vi "IDEX FGV.vi"(7 "Function":T2(ring), 8 "error in":errorcluster, 9 "Command":string, 10 "Position":T1(ring), 11 "VISA resource name":refnum<visa-resource-name>) -> (0 "error out":errorcluster, 3 "Read String":string)   [LabVIEW 2019, in "IDEX.lvlib"]
uses:
  IDEX.lvlib
  <vilib>/Instr/_visa.llb/VISA Configure Serial Port (Instr).vi
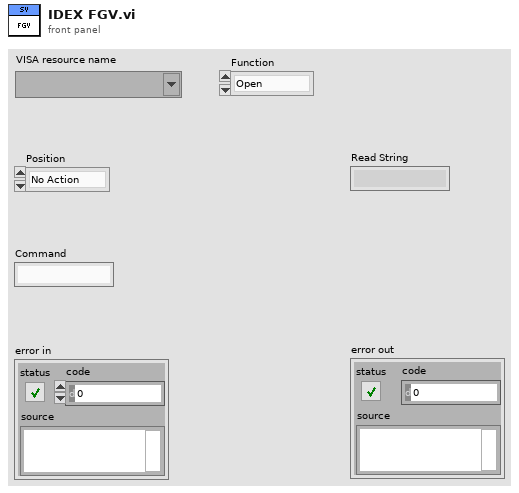
[diagram p1: front panel]
types:
  T1 = enum16{"No Action", "Position 1", "Position 2", "Position 3", "Position 4", "Position 5", "Position 6"}
  T2 = enum16{"Open", "Read", "Move", "Home", "Command", "Close"}
  T3 = cluster{"VISA resource":refnum<visa-resource-name>, "Read String":string}
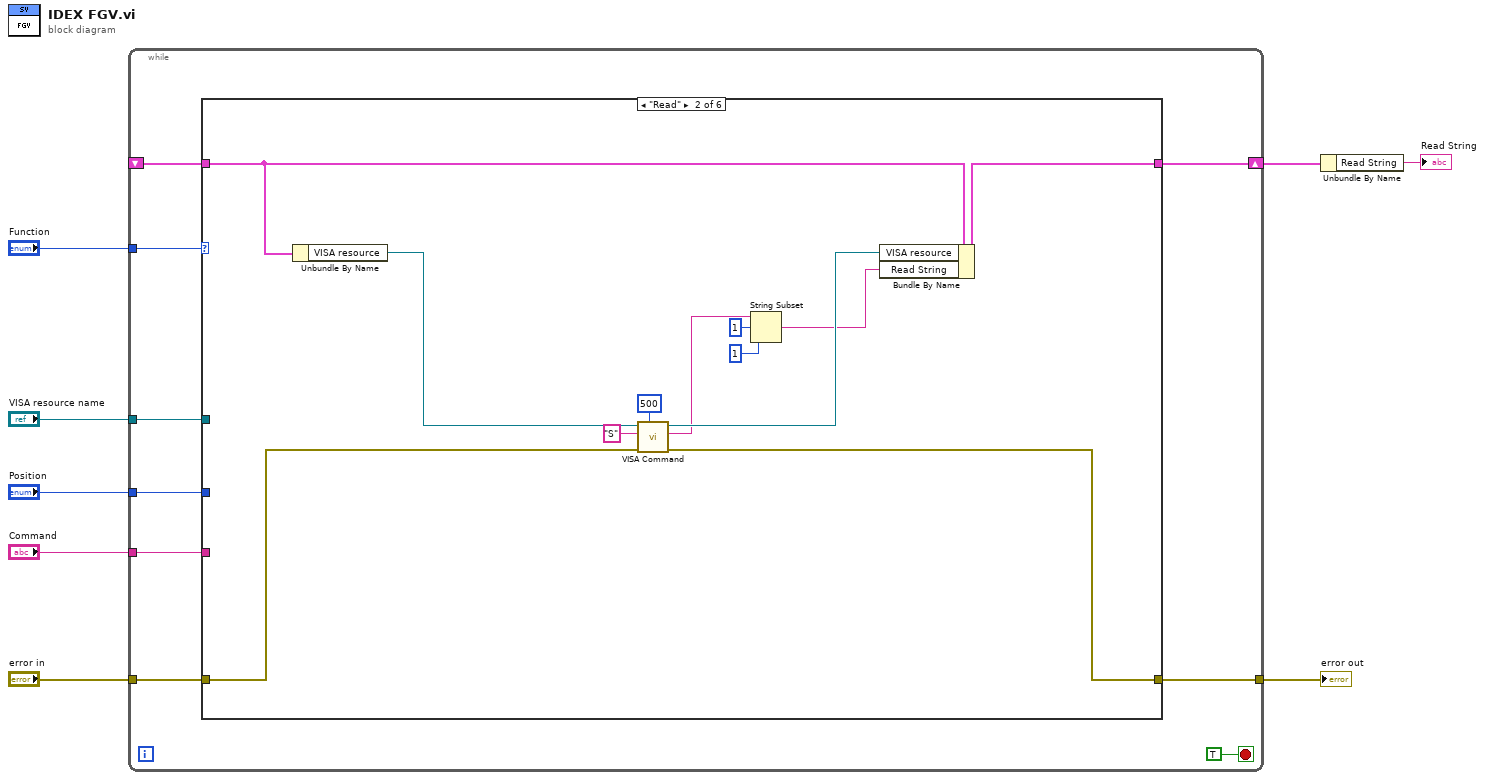
[diagram p0: block diagram]
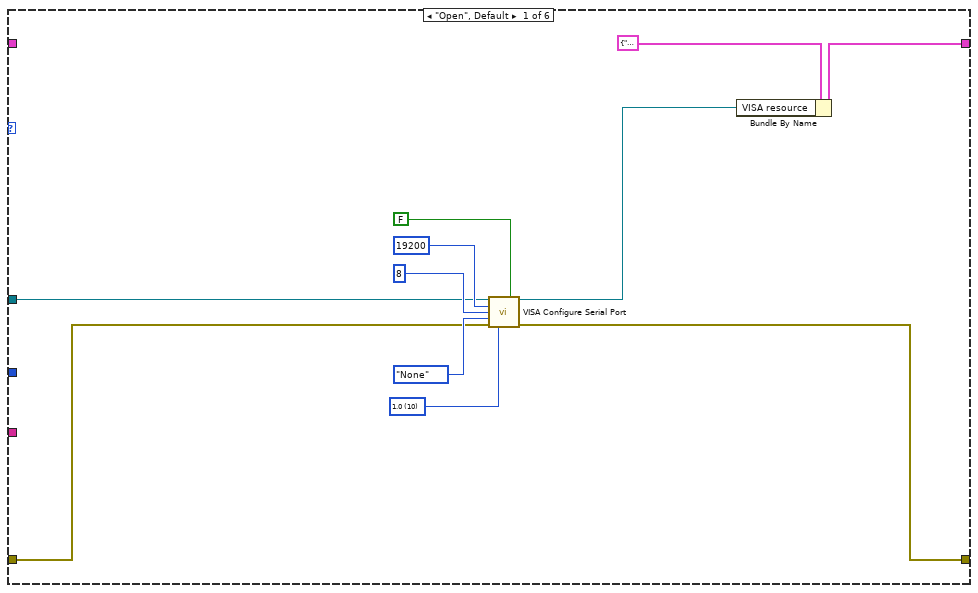
[diagram p2: hidden frame]
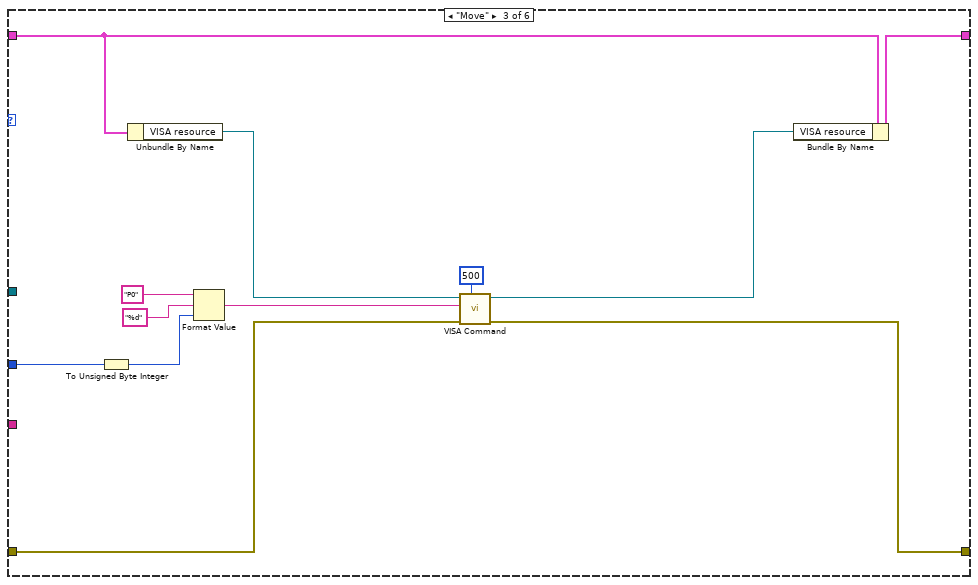
[diagram p3: hidden frame]
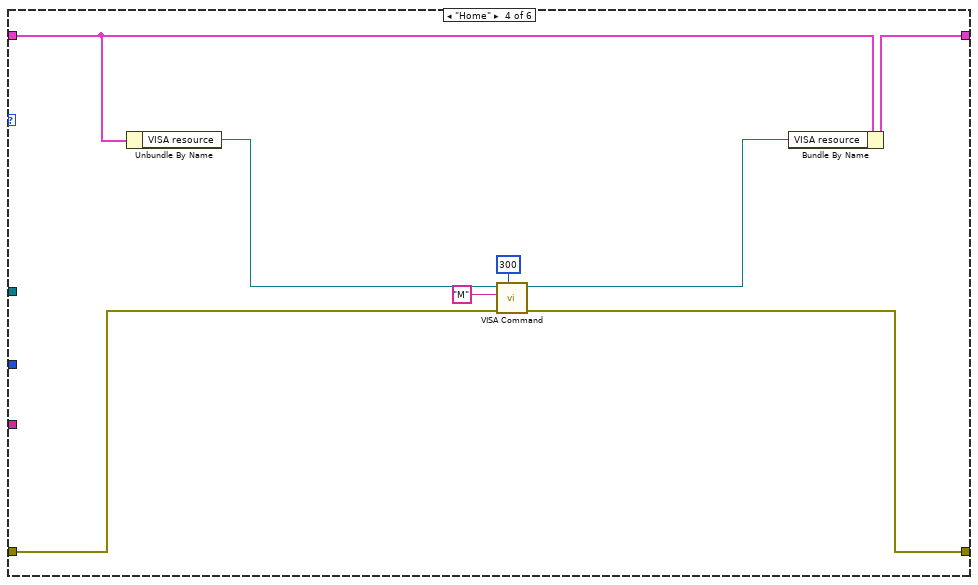
[diagram p4: hidden frame]
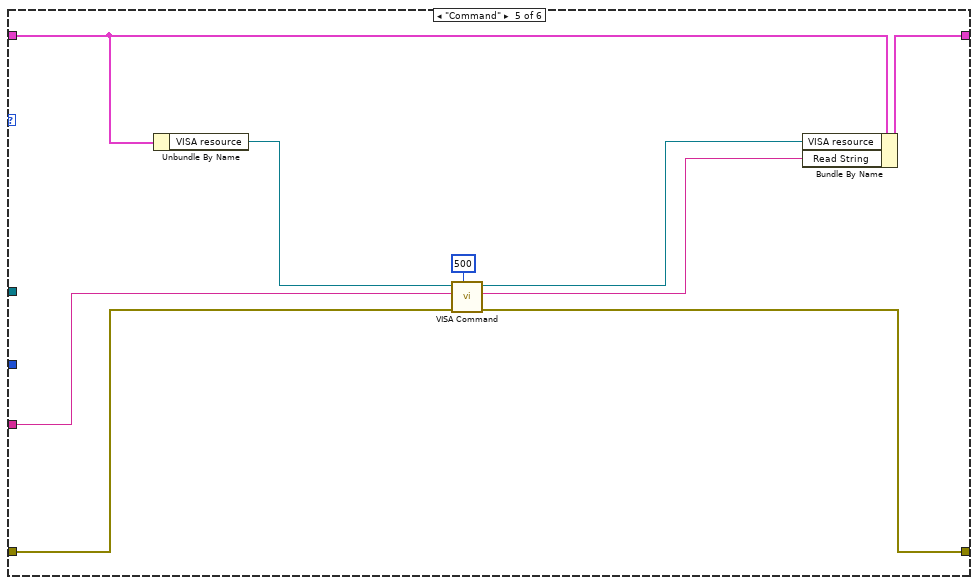
[diagram p5: hidden frame]
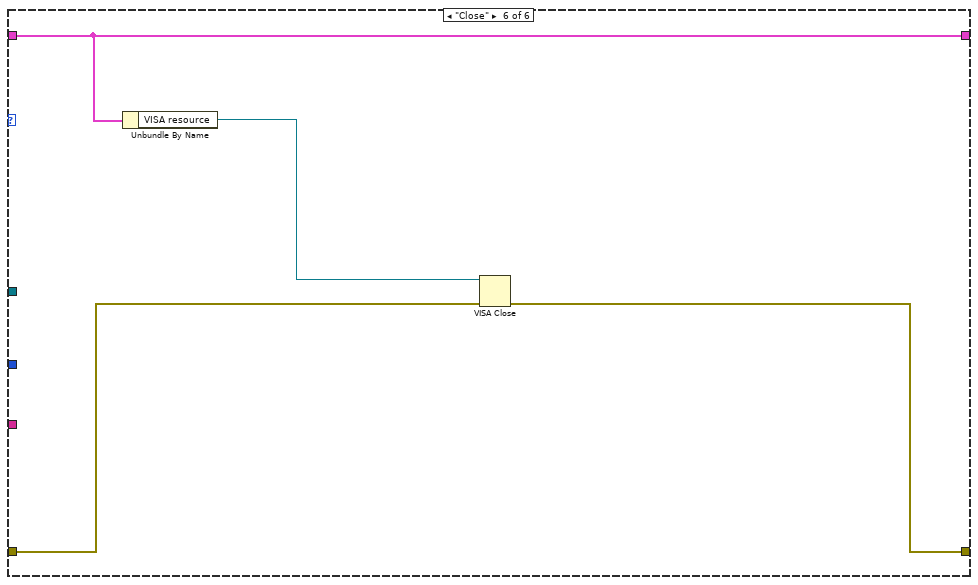
[diagram p6: hidden frame]
diagram:
  n1 = while {
    shift-right: [w15] -> w2
    shift-left: _ -> [w16]
    tunnel: "Function" -> [w14]
    tunnel: "error in" -> [w13]
    tunnel: [w9] -> w6
    tunnel: "VISA resource name" -> [w12]
    tunnel: "Command" -> [w11]
    tunnel: "Position" -> [w10]
    stop <- TRUE stop-if-true
    n2 = case shown="\"Read\"" w14 {
      tunnel: w16 -> [_ w37 w46 w58 w66 w73]
      tunnel: [w19 w35 w42 w54 w64 w73] -> w15
      tunnel: w13 -> [w22 w40 w45 w60 w68 w72]
      tunnel: [w21 w33 w43 w59 w67 w70] -> w9
      tunnel: w12 -> [w23 _ _ _ _ _]
      tunnel: w11 -> [_ _ _ _ w69 _]
      tunnel: w10 -> [_ _ w50 _ _ _]
      frame "Open", Default {
        w26 = u16 10 items=["1.0"=10, "1.5"=15, "2.0"=20] ("stop bits (10: 1 bit)")
        n3 = call-poly "VISA Configure Serial Port"("VISA resource name"=w23, "Enable Termination\nChar (T)"=FALSE ("Enable Termination\nChar (T)"), "baud rate (9600)"=u32 19200, "data bits (8)"=u16 8, "parity (0:none)"=enum16{"None", "Odd", "Even", "Mark", "Space"}."None", "error in (no error)"=w22, "stop bits (10: 1 bit)"=w26) -> ("VISA resource name out"=w18:refnum<visa-resource-name>, "error out"=w21:errorcluster)  [unwired: 7 in]
        n4 = Bundle By Name(cluster=T3 {"VISA resource"="", "Read String"=""}, "VISA resource"=w18) -> (w19:T3)
      }
      frame "Read" {
        n5 = Unbundle By Name(w37) -> ("VISA resource"=w36:refnum<visa-resource-name>)
        n6 = call "VISA Command.vi"("Wait (ms)"=u32 500, "error in (no error)"=w40, "Command"="S", "VISA resource name"=w36) -> ("error out"=w33:errorcluster, "read buffer"=w32:string, "VISA resource name out"=w34:refnum<visa-resource-name>)  [unwired: 5 in]
        n7 = String Subset(string=w32, offset (0)=1, length (rest)=1 ("length (rest)")) -> (substring=w29:string)
        n8 = Bundle By Name(cluster=w37, "VISA resource"=w34, "Read String"=w29) -> (w35:T3)
      }
      frame "Move" {
        n9 = To Unsigned Byte Integer(number=w50) -> (unsigned 8bit integer=w49:u8)
        n10 = Unbundle By Name(w46) -> ("VISA resource"=w44:refnum<visa-resource-name>)
        n11 = Format Value(string ("")="P0", format string="%d", value (0)=w49) -> (output string=w48:string)
        n12 = call "VISA Command.vi"("Wait (ms)"=u32 500, "error in (no error)"=w45, "Command"=w48, "VISA resource name"=w44) -> ("error out"=w43:errorcluster, "VISA resource name out"=w41:refnum<visa-resource-name>)  [unwired: 5 in, 1 out]
        n13 = Bundle By Name(cluster=w46, "VISA resource"=w41) -> (w42:T3)
      }
      frame "Home" {
        n14 = Unbundle By Name(w58) -> ("VISA resource"=w55:refnum<visa-resource-name>)
        n15 = call "VISA Command.vi"("Wait (ms)"=u32 300, "error in (no error)"=w60, "Command"="M", "VISA resource name"=w55) -> ("error out"=w59:errorcluster, "VISA resource name out"=w53:refnum<visa-resource-name>)  [unwired: 5 in, 1 out]
        n16 = Bundle By Name(cluster=w58, "VISA resource"=w53) -> (w54:T3)
      }
      frame "Command" {
        n17 = Unbundle By Name(w66) -> ("VISA resource"=w65:refnum<visa-resource-name>)
        n18 = call "VISA Command.vi"("Wait (ms)"=u32 500, "error in (no error)"=w68, "Command"=w69, "VISA resource name"=w65) -> ("error out"=w67:errorcluster, "read buffer"=w62:string, "VISA resource name out"=w63:refnum<visa-resource-name>)  [unwired: 5 in]
        n19 = Bundle By Name(cluster=w66, "VISA resource"=w63, "Read String"=w62) -> (w64:T3)
      }
      frame "Close" {
        n20 = Unbundle By Name(w73) -> ("VISA resource"=w71:refnum<visa-resource-name>)
        n21 = VISA Close(VISA resource name=w71, error in (no error)=w72) -> (error out=w70:errorcluster)
      }
    }
  }
  "error out" <- w6
  n22 = Unbundle By Name(w2) -> ("Read String"=→"Read String":string)
